vi "decodeMap.vi"(8 "error in (no error)":errorcluster, 10 "ByteArray":u8[](array[numeric]) format="%.0x") -> (0 "error out":errorcluster, 2 "variant":variant, 3 "ByteArray":u8[](array[numeric]), 5 "Type":string)   [LabVIEW 2016, in "MsgPack.lvlib"]
uses:
  MsgPack.lvlib
  <vilib>/Utility/error.llb/Error Cluster From Error Code.vi
  <vilib>/ErrorRing/Error Ring.xnode
panel:
  out "Array":string[](array[string])
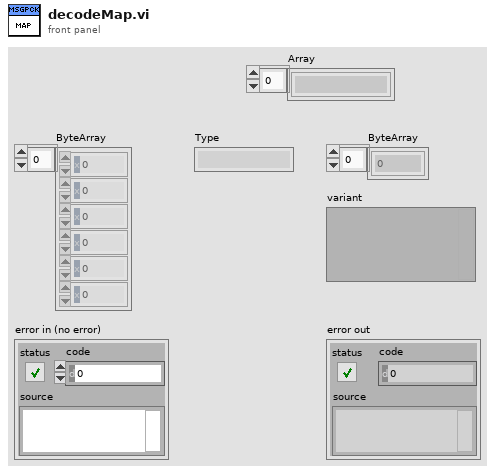
[diagram p1: front panel]
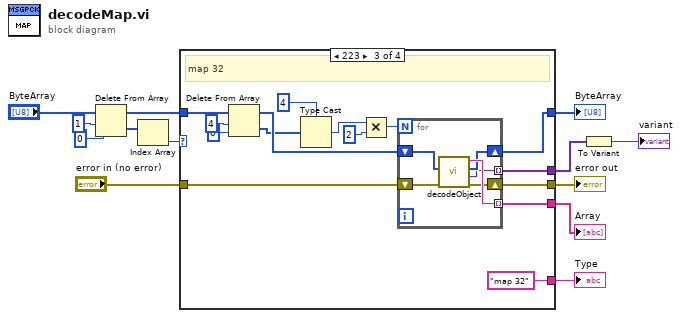
[diagram p0: block diagram]
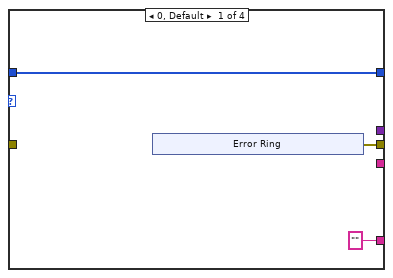
[diagram p2: hidden frame]
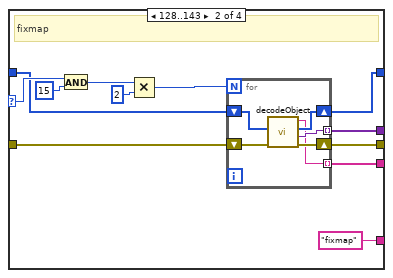
[diagram p3: hidden frame]
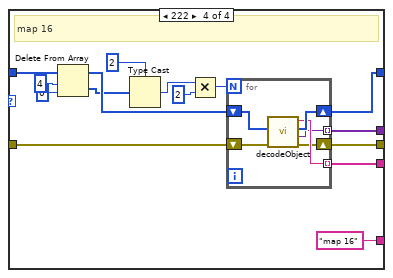
[diagram p4: hidden frame]
diagram:
  n1 = Delete From Array(array="ByteArray", length=1, index=0) -> (deleted portion=w4:u8[], array with subset deleted=w3:u8[])
  n2 = Index Array(array=w4) -> (element=w10:u8)  [unwired: 1 in]
  n3 = case shown="223" w10 {
    selector: w10 -> [_ w32 _ _]
    tunnel: [w16 w28 w52 w73] -> w12
    tunnel: "error in (no error)" -> [_ w29 w53 w74]
    tunnel: ["" "fixmap" "map 32" "map 16"] -> w9
    tunnel: [_ w27 w51 w72] -> w8
    tunnel: w3 -> [w14 w30 w49 w70]
    tunnel: [_ w26 w50 w71] -> w7
    tunnel: [w14 w25 w44 w65] -> w2
    frame 0, Default {
      n4 = xnode "Error Ring"() -> ("Fehler (Ausgang)"=w16:errorcluster)
    }
    frame 128..143 {
      # "fixmap"
      n5 = And(x=w32, y=u8 15) -> (x .and. y?=w23:u8)
      n6 = Multiply(x=w23, y=u8 2) -> (x*y=w22:u8)
      n7 = for {
        N: w22 -> [_]
        shift-right: [w36] -> w25
        shift-left: w30 -> [w34]
        tunnel: [w35] -> w26 mode=indexing
        shift-right: [w38] -> w28
        shift-left: w29 -> [w39]
        tunnel: [w37] -> w27 mode=indexing
        n8 = call "decodeObject.vi"("error in (no error)"=w39, "ByteArray"=w34) -> ("error out"=w38:errorcluster, "Variant"=w37:variant, "RemainingBytes"=w36:u8[], "Type"=w35:string)  [unwired: 6 in]
      }
    }
    frame 223 {
      # "map 32"
      n9 = Delete From Array(array=w49, length=4, index=0) -> (deleted portion=w46:u8[], array with subset deleted=w47:u8[])
      n10 = Type Cast(type=u32 4 ("length"), x=w46) -> (*(type *) &x=w42:u32)
      n11 = Multiply(x=w42, y=u8 2) -> (x*y=w41:u32)
      n12 = for {
        N: w41 -> [_]
        shift-right: [w57] -> w44
        shift-left: w47 -> [w59]
        tunnel: [w58] -> w50 mode=indexing
        shift-right: [w55] -> w52
        shift-left: w53 -> [w60]
        tunnel: [w56] -> w51 mode=indexing
        n13 = call "decodeObject.vi"("error in (no error)"=w60, "ByteArray"=w59) -> ("error out"=w55:errorcluster, "Variant"=w56:variant, "RemainingBytes"=w57:u8[], "Type"=w58:string)  [unwired: 6 in]
      }
    }
    frame 222 {
      # "map 16"
      n14 = Delete From Array(array=w70, length=4, index=0) -> (deleted portion=w67:u8[], array with subset deleted=w68:u8[])
      n15 = Type Cast(type=u32 2 ("length"), x=w67) -> (*(type *) &x=w63:u32)
      n16 = Multiply(x=w63, y=u8 2) -> (x*y=w62:u32)
      n17 = for {
        N: w62 -> [_]
        shift-right: [w80] -> w65
        shift-left: w68 -> [w81]
        tunnel: [w79] -> w71 mode=indexing
        shift-right: [w77] -> w73
        shift-left: w74 -> [w76]
        tunnel: [w78] -> w72 mode=indexing
        n18 = call "decodeObject.vi"("error in (no error)"=w76, "ByteArray"=w81) -> ("error out"=w77:errorcluster, "Variant"=w78:variant, "RemainingBytes"=w80:u8[], "Type"=w79:string)  [unwired: 6 in]
      }
    }
  }
  "error out" <- w12
  "Type" <- w9
  "Array" <- w7
  "ByteArray" <- w2
  n19 = To Variant(anything=w8) -> (Variant=→"variant":variant)
